vi "strain_gauge_run.vi"(8 "error in":errorcluster, 10 "Samples per Loop":i32=100, 11 "task/channels in":refnum<k21>) -> (0 "error out":errorcluster, 2 "Waveform Chart":waveform(dbl)[](graph), 3 "task out":refnum<k21>)   [LabVIEW 2022 SP3]
uses:
  <vilib>/DAQmx/read.llb/DAQmx Read (Analog 1D Wfm NChan NSamp).vi
  <vilib>/DAQmx/miscellaneous.llb/DAQmx Fill In Error Info.vi
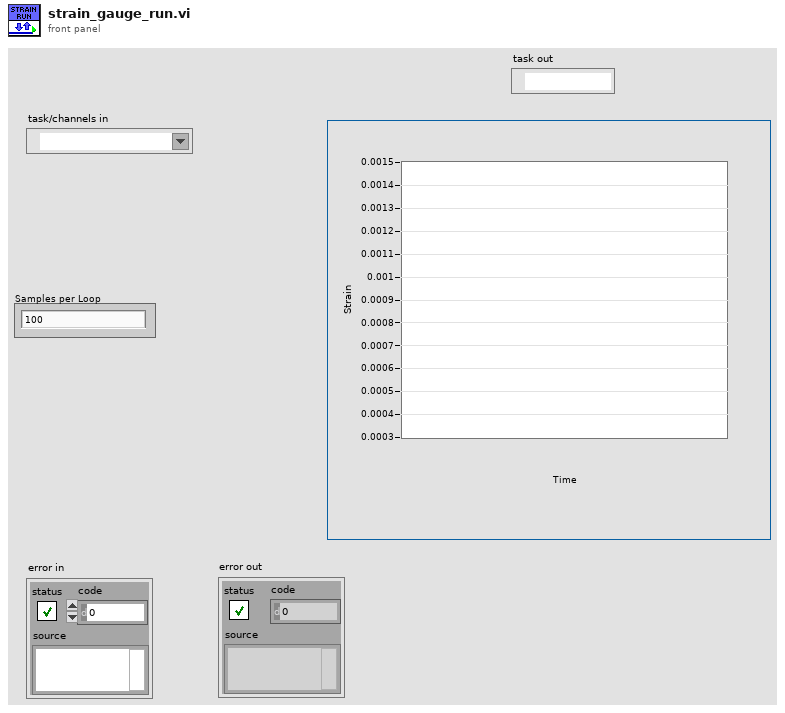
[diagram p1: front panel]
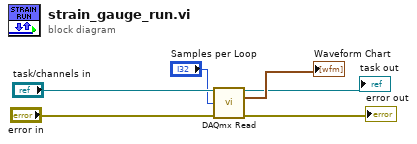
[diagram p0: block diagram]
diagram:
  n1 = call-poly <vilib>:"DAQmx Read.vi"("task/channels in"="task/channels in", "number of samples per channel"="Samples per Loop", "error in"="error in") -> ("task out"=→"task out":refnum<k21>, "data"=→"Waveform Chart":waveform(dbl)[], "error out"=→"error out":errorcluster)  [unwired: 10 in]
